vi "ExSubCreateImage.vi"(2 "error in (no error)":errorcluster, 5 "Camera Handle":u32) -> (0 "error out":errorcluster, 1 "Handles Out":T1)   [LabVIEW 2010]
panel:
  # "ExSubCreateFileImage:\nThis is a SubVI that creates a file, and image \nobjects and returns the handles bundled in a cluster \nthat includes a pulser and camera handle"
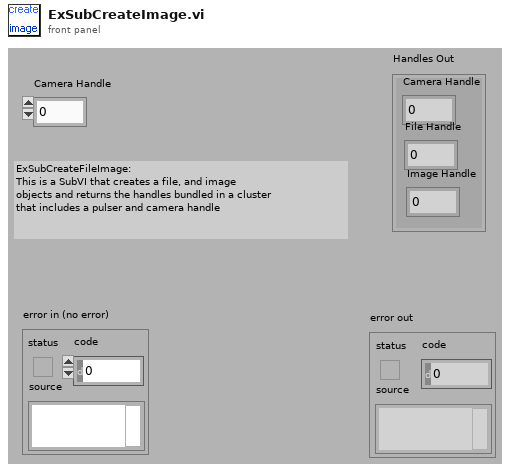
[diagram p1: front panel]
types:
  T1 = cluster{"Camera Handle":u32, "File Handle":u32, "Image Handle":u32}
  T2 = cluster{"Camera Handle":u32, i32, "Image Handle":u32}
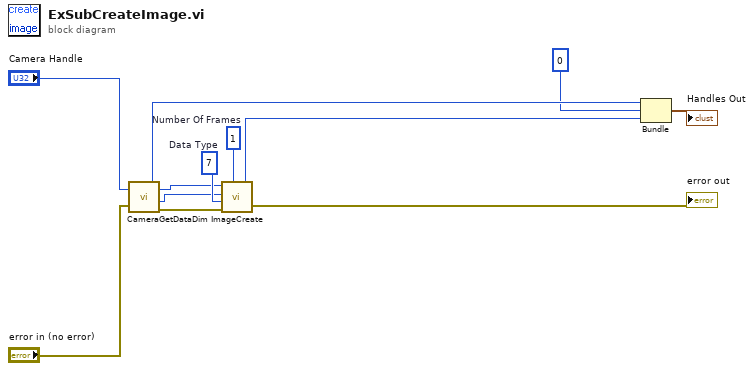
[diagram p0: block diagram]
diagram:
  w6 = u32 1  # Number Of Frames
  w7 = u32 7  # Data Type
  n1 = call <userlib>:"CameraGetDataDim.vi"("Camera Handle"="Camera Handle", "error in"="error in (no error)") -> ("Camera Handle"=w9:u32, "Xdim"=w4:u32, "Ydim"=w5:u32, "error out"=w12:errorcluster)
  n2 = call <userlib>:"ImageCreate.vi"("X dimension"=w4, "Y dimension"=w5, "Data Type"=w7, "error in"=w12, "Number Of Frames"=w6) -> ("Image Handle"=w8:u32, "error out"=→"error out":errorcluster)
  n3 = Bundle("Camera Handle"=w9, 0, "Image Handle"=w8) -> (→"Handles Out":T2)  [unwired: 1 in]
